vi "CMD StopDaq.vi"(8 "error in (no error)":errorcluster, 11 "DAQ in":refnum<class "DAQ.lvclass">) -> (0 "error out":errorcluster, 3 "DAQ out":refnum<class "DAQ.lvclass">)   [LabVIEW 2017, in "DAQ.lvclass"]
doc: "Developed by Kevin Thompson\nkevin@thompsonengineering.net\n\nCopyright 2018-2020\nThompson Engineering, LLC"
uses:
  DAQ.lvclass
  DataTypes/AsyncCmd_DAQ--enum.ctl
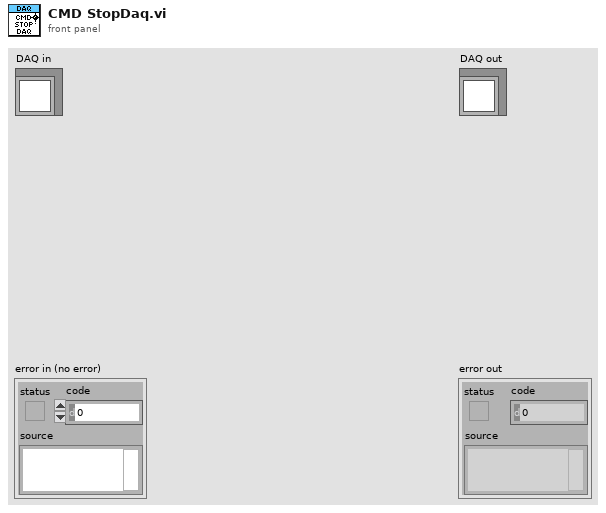
[diagram p1: front panel]
types:
  T1 = typedef "DAQ.lvclass/AsyncCmd_DAQ--enum.ctl" = enum16{"StartDAQ", "StopDAQ", "CfgDAQ"}
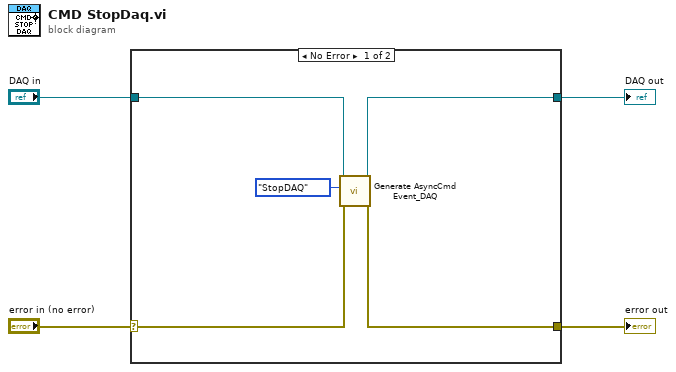
[diagram p0: block diagram]
diagram:
  n1 = case shown="No Error" "error in (no error)" {
    selector: "error in (no error)" -> [w9 w11]
    tunnel: [w8 w11] -> w3
    tunnel: [w6 w10] -> w1
    tunnel: "DAQ in" -> [w7 w10]
    frame No Error {
      n2 = call "Generate AsyncCmd Event_DAQ.vi"("error in (no error)"=w9, "AsyncCmd"=AsyncCmd_DAQ--enum."StopDAQ" ("AsyncMsg"), "DAQ"=w7) -> ("error out"=w8:errorcluster, "DAQ out"=w6:refnum<class "DAQ.lvclass">)  [unwired: 7 in]
    }
    frame Error {
    }
  }
  "error out" <- w3
  "DAQ out" <- w1
